vi "point_line_distance.vi"(9 "Point":T1, 10 "Line":T2) -> (2 "Distance":sgl)   [LabVIEW 2020, in "3DPC_SurfacePlot.xctl"]
uses:
  <vilib>/Native 3D Graph/xcontrol/3DPC_SurfacePlot.xctl
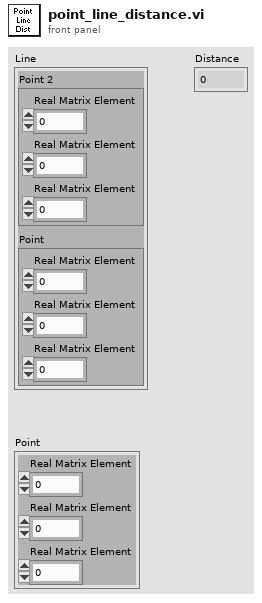
[diagram p1: front panel]
types:
  T1 = cluster{"Real Matrix Element":dbl, "Real Matrix Element":dbl, "Real Matrix Element":dbl}
  T2 = cluster{"Point 2":cluster{"Real Matrix Element":dbl, "Real Matrix Element":dbl, "Real Matrix Element":dbl}, "Point":cluster{"Real Matrix Element":dbl, "Real Matrix Element":dbl, "Real Matrix Element":dbl}}
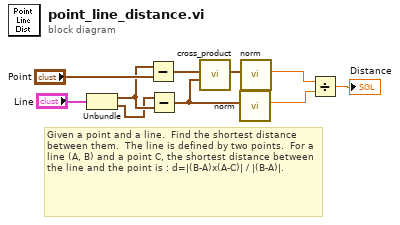
[diagram p0: block diagram]
diagram:
  # "Given a point and a line.  Find the shortest distance between them.  The line is defined by two points.  For a line (A, B) and a point C, the shortest distance between the line and the point is : d=|(B-A)x(A-C)| / |(B-A)|."
  n1 = Unbundle("Line") -> ("Point 2"=w2:T1, "Point"=w1:T1)
  n2 = Subtract(x=w2, y="Point") -> (x-y=w5:T1)
  n3 = Subtract(x=w1, y=w2) -> (x-y=w4:T1)
  n4 = call <vilib>:"cross_product.vi"("Vect 2"=w4, "Vect 1"=w5) -> ("Vect Out"=w9:cluster{"X":sgl, "Y":sgl, "Z":sgl})  [unwired: 1 in, 8 out]
  n5 = call <vilib>:"norm.vi"("Vector"=w4) -> ("Norm"=w7:sgl)  [unwired: 10 out]
  n6 = call <vilib>:"norm.vi"("Vector"=w9) -> ("Norm"=w8:sgl)  [unwired: 10 out]
  n7 = Divide(x=w8, y=w7) -> (x/y=→"Distance":sgl)
